vi "New TA Binding.vi"(8 "error in (no error)":errorcluster, 10 "Index (out of array range means creating new)":i32, 11 "Motions in":refnum<class "Motions.lvclass">) -> (0 "error out":errorcluster, 2 "New TA Binding out":T1, 3 "Motions out":refnum<class "Motions.lvclass">)   [LabVIEW 2016, in "Hardware.lvlib" / "Motions.lvlib" / "Motions.lvclass"]
uses:
  <userlib>/Common Components/Hardware/Abstract System/Motions/Motions/Motions.lvclass
  <userlib>/TSPopup/TSPopup.Popup Cluster.ctl
  <userlib>/Common Components/Hardware/Abstract System/Motions/Motions/TA Binding Data.ctl
  <userlib>/Common Components/Hardware/Abstract System/Motions/Motions/Motions.lvclass/Motions.ctl
  <userlib>/Common Components/Hardware/Abstract Hardware/Hardware.lvclass/Hardware.ctl
  <userlib>/TSPopup/TSPopup.Popup Call Parameters.ctl
  <userlib>/TSPopup/TSPopup.Data Type.ctl
  <userlib>/TSPopup/TSPopup.lvclass
  <userlib>/TSPopup/TSPopup.Grid.Cell Info.ctl
  <userlib>/Common Components/Hardware/Abstract Hardware/Read Label.vi
  <userlib>/Common Components/Hardware/Motor/Motor/Motor.lvclass
  C:/Program Files (x86)/National Instruments/LabVIEW 2016/user.lib/Common Components/Hardware/Abstract Hardware/Hardware.lvclass
panel:
  in  "Triggers for Array OR":T2(array[cluster]) {"Triggers for Array AND"."Motor" items=["X", "Y", "Z", "R1", "R3"]}
  in  "Popups":T3 {"Boolean" items=["False", "True"]; "Ring" items=["Enable Motor", "Disable Motor", "Move Motor"]}
  in  "Actions":i32(listbox)
  # "OR"
  # "AND"
  # "Type Sensitive\nPopup"
  # "Boolean Colors"
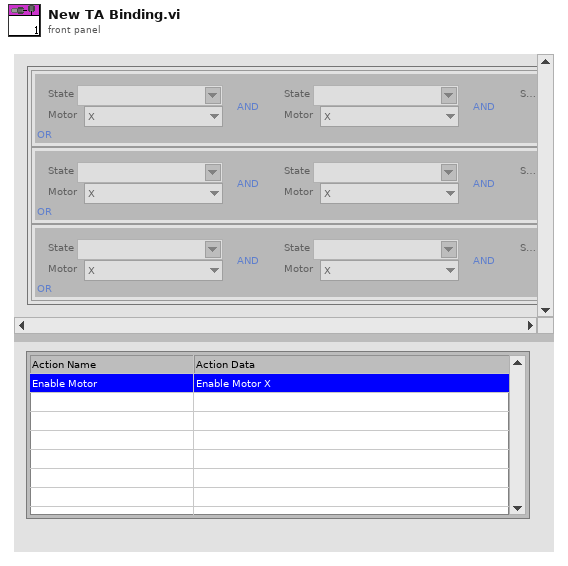
[diagram p1: front panel]
types:
  T1 = typedef "Hardware.lvlib/Motions.lvlib/Motions.lvclass/TA Binding Data.ctl" = cluster{"Triggers":cluster{"Triggers for Array AND":cluster{"Index":u8, "State Name":string}[]}[], "Actions":cluster{"Action Name":string, "Action Data":string}[]}
  T2 = cluster{"Triggers for Array AND":cluster{"Motor":u16, "State":string}[]}[]
  T3 = typedef "TSPopup.lvlib/TSPopup.lvclass/TSPopup.Popup Cluster.ctl" = cluster{"Unknown":bool, "Unknown 2":bool, "String":string, "Integer":i32, "Float":dbl, "Color":u32, "Boolean":u32, "Ring":u32, "Captioned String":cluster{"String":string, "OK":bool, "Cancel":bool}, "Captioned Integer":cluster{"First":i32, "OK":bool, "Cancel":bool}, "Boolean Colors":cluster{"False":cluster{"FG":u32, "BG":u32}, "True":cluster{"FG":u32, "BG":u32}, "T  to  F":cluster{"FG":u32, "BG":u32}, "F  to  T":cluster{"FG":u32, "BG":u32}, "OK":bool, "Cancel":bool}, "2-Int Cluster":cluster{"First":i32, "Second":i32, "OK":bool, "Cancel":bool}, "4-Int Cluster":cluster{"First":i32, "Second":i32, "Third":i32, "Fourth":i32, "OK":bool, "Cancel":bool}, "check":bool}
  T4 = cluster{"Action Name":string, "JSON info":cluster{"path":string, "data type":enum16{"INT", "DBL", "BOOL", "String"}}[], "String Format":string}[]
  T5 = cluster{"Data Types":cluster{"Data Type":string, "Ring Strings":string[]}[]}[]
  T6 = typedef "TSPopup.lvlib/TSPopup.lvclass/TSPopup.Data Type.ctl" = enum16{"Unkown", "NO POPUP", "String", "Integer", "Float", "Color", "Boolean", "Ring", "Captioned String", "Captioned Integer", "Button Color", "2 Int Cluster", "4 Int Cluster", "check"}
  T7 = typedef "TSPopup.lvlib/TSPopup.lvclass/TSPopup.Popup Call Parameters.ctl" = cluster{"Prop Type":T6, "Initial Value":variant, "Caption Strings":string[], "Ring Strings":string[], "Cell Rect":cluster{"left":i16, "top":i16, "right":i16, "bottom":i16}, "Mouse Coords":cluster{"x":i16, "y":i16}, "Call Data":variant}
  T8 = typedef "TSPopup.lvlib/TSPopup.lvclass/TSPopup.Grid.Cell Info.ctl" = cluster{"Tag":string, "Row":i32, "Column":i32, "In Symbol?":bool, "In Data?":bool, "Cell String":string, "Ctl Refnum":refnum<vi>, "Prop Type":T6, "Ring Strings":string[]}
  T9 = cluster{"Data Type":string, "Ring Strings":string[]}[]
  T10 = cluster{"Data Types":cluster{"Data Type":string, "Ring Strings":string[]}[]}
  T11 = typedef "LVPoint32TypeDef.ctl" = cluster{"Horizontal":i32, "Vertical":i32}
  T12 = typedef "LVRowAndColumnTypeDef.ctl" = cluster{"Row":i32, "Column":i32}
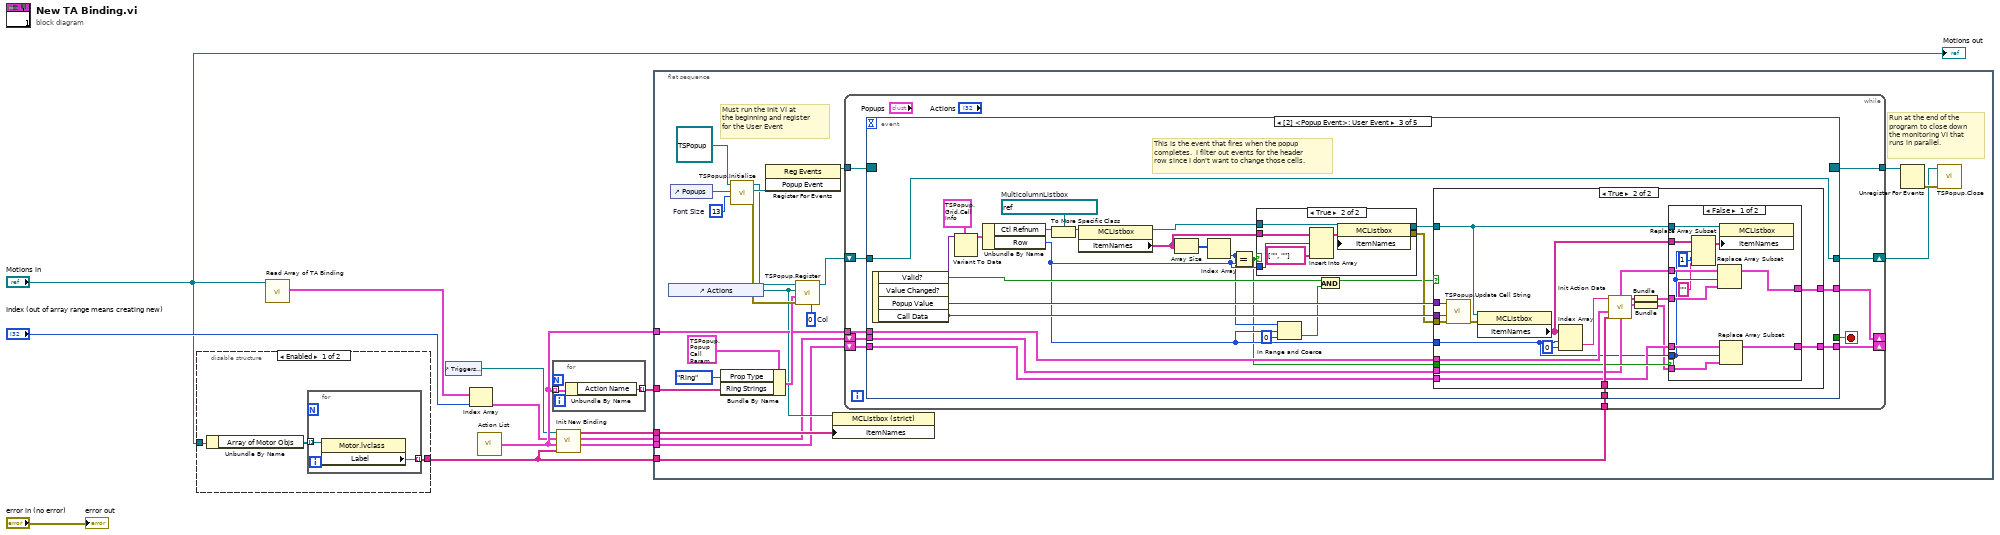
[diagram p0: block diagram]
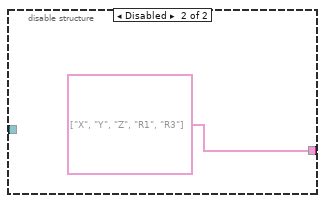
[diagram p2: hidden frame]
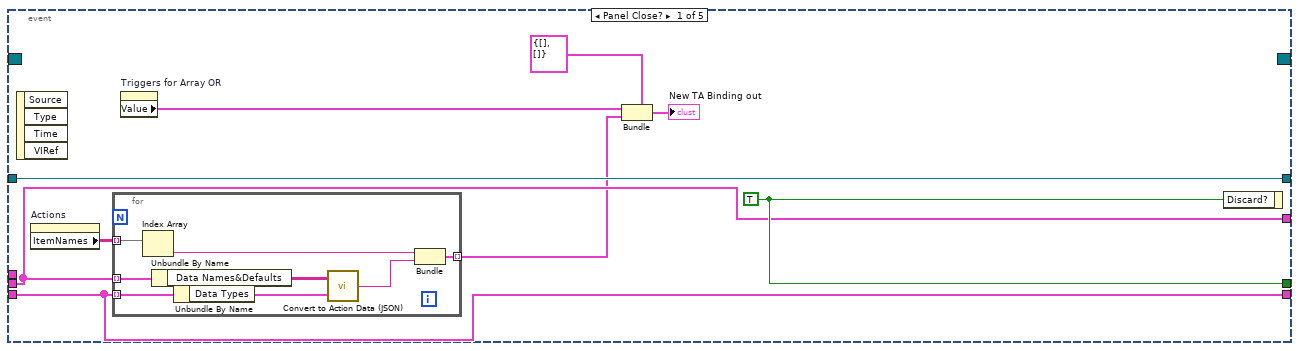
[diagram p3: hidden frame]
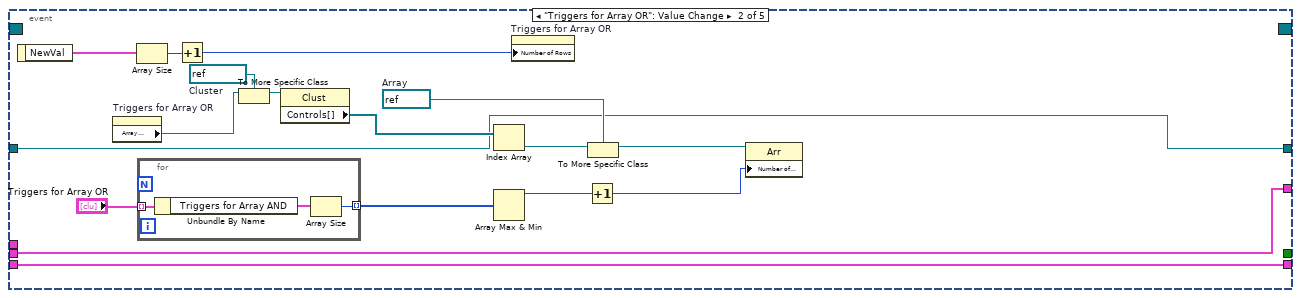
[diagram p4: hidden frame]
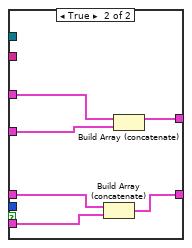
[diagram p7: hidden frame]
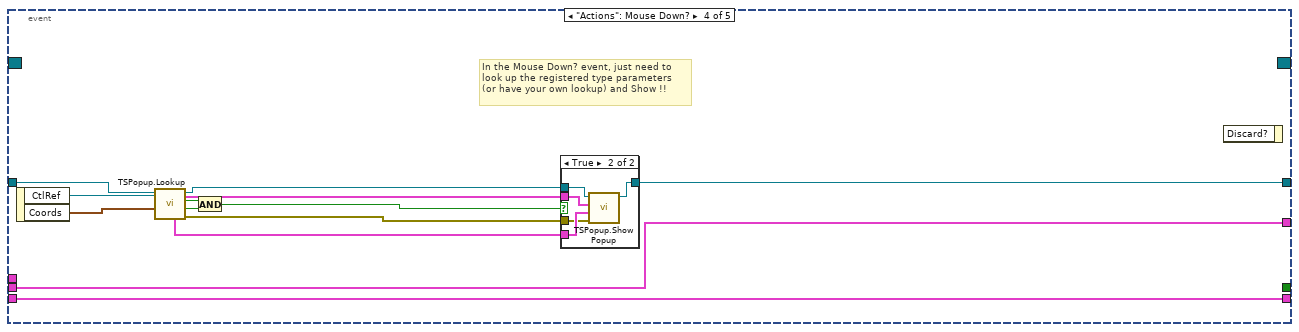
[diagram p8: hidden frame]
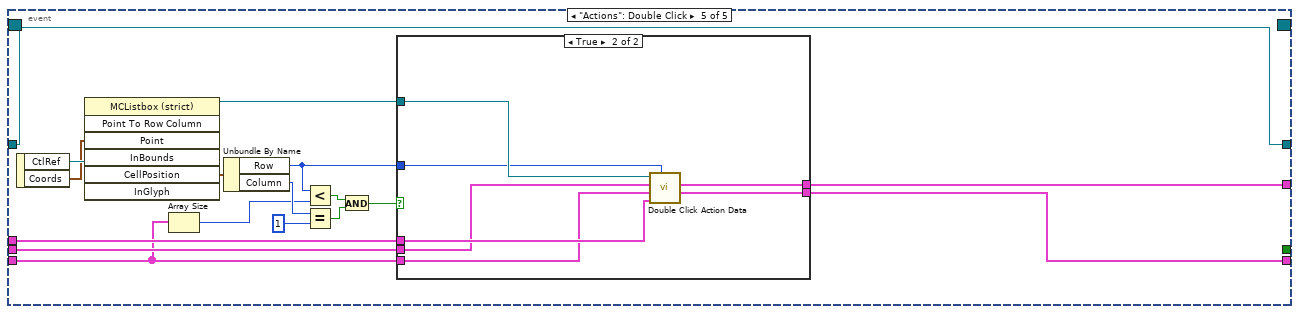
[diagram p10: hidden frame]
diagram:
  n1 = disable-structure shown="Enabled" {
    disable-tunnel: "Motions in" -> [w15 _]
    disable-tunnel: [w13 string[] ["X", "Y", "Z", "R1", "R3"]] -> w2
    frame Enabled {
      n2 = Unbundle By Name(w15) -> ("Array of Motor Objs"=w14:refnum<class "Motor.lvclass">[])
      n3 = for {
        tunnel: w14 -> [w17] mode=indexing
        tunnel: [w16] -> w13 mode=indexing
        n4 = property class="Motor.lvclass"(reference=w17) -> ("Label"=w16:string)  [unwired: 1 in, 2 out]
      }
    }
    frame Disabled {
    }
  }
  n5 = call <userlib>:"Read Array of TA Binding.vi"("Motions in"="Motions in") -> ("Array of TA Binding"=w9:T1[])  [unwired: 9 in, 1 out]
  n6 = control-ref of="Triggers for Array OR"() -> (w7:refnum<vi>)
  n7 = Index Array(array=w9, index="Index (out of array range means creating new)") -> (element=w5:T1)
  n8 = call <userlib>:"Action List.vi"() -> ("Action List"=w11:T4)
  n9 = for {
    tunnel: w11 -> [w20] mode=indexing
    tunnel: [w19] -> w12 mode=indexing
    n10 = Unbundle By Name(w20) -> ("Action Name"=w19:string)
  }
  n11 = call <userlib>:"Init New Binding.vi"("Motor Labels"=w2, "Action List"=w11, "TriggerAction Cluster"=w5, "Triggers Arr Ref"=w7) -> ("Array of Data Types"=w3:T5, "Array of Data Names&Defaults"=w4:cluster{"Data Names&Defaults":string[][]}[], "2-col Arr Actions out"=w6:string[][])  [unwired: 5 in]
  n12 = flat-sequence {
    tunnel: w12 -> [w27]
    tunnel: w11 -> [w26]
    tunnel: w6 -> [w25]
    tunnel: w4 -> [w23]
    tunnel: w3 -> [w22]
    tunnel: w2 -> [w21]
    frame #0 {
      w36 = 0  # Col
      w42 = u32 13  # Font Size
      # "Run at the end of the\nprogram to close down\nthe monitoring VI that\nruns in parallel."
      # "Must run the Init VI at\nthe beginning and register\nfor the User Event"
      n13 = control-ref of="Actions"() -> (w24:refnum<vi>)
      n14 = control-ref of="Popups"() -> (w28:refnum<vi>)
      n15 = Bundle By Name(cluster=T7 {"Prop Type"=enum."Unkown", "Initial Value"=variant, "Caption Strings"=[], "Ring Strings"=[], "Cell Rect"={"left"=0, "top"=0, "right"=0, "bottom"=0}, "Mouse Coords"={"x"=0, "y"=0}, "Call Data"=variant} ("Show Popup (type only)"), "Prop Type"=TSPopup.Data_Type."Ring", "Ring Strings"=w27) -> (w33:T7)
      n16 = call <userlib>:"TSPopup.Initialize.vi"("Font Size"=w42, "Popup Cluster Ref"=w28, "TSPopup in"=refnum<class "TSPopup.lvclass"> refnum) -> ("error out"=w37:errorcluster, "Popup Event"=w41:refnum<user-event>, "TSPopup out"=w31:refnum<class "TSPopup.lvclass">)  [unwired: 6 in]
      n17 = register-events(w41) -> (reference out=w40:refnum<event-registration>)  [unwired: 2 in, 1 out]
      n18 = call <userlib>:"TSPopup.Register.vi"("Col (unwired = all columns)"=w36, "error in (no error)"=w37, "Parameters"=w33, "Ctl Refnum"=w24, "TSPopup in"=w31) -> ("TSPopup out"=w30:refnum<class "TSPopup.lvclass">)  [unwired: 4 in, 2 out]
      n19 = property on="Property Node" class="MCListbox (strict)"(reference=w24, "ItemNames"=w25) -> ()  [unwired: 1 in, 2 out]
      n20 = while {
        tunnel: w40 -> [w53]
        tunnel: [w52] -> w39
        shift-right: [w49] -> w29
        shift-left: w30 -> [w50]
        tunnel: w26 -> [w48]
        shift-right: [w44] -> _
        shift-left: w23 -> [w47]
        shift-right: [w45] -> _
        shift-left: w22 -> [w46]
        tunnel: w21 -> [w43]
        stop <- w51 stop-if-true
        n21 = event shown="[2] <Popup Event>: User Event" {
          selector: w53 -> [_ _ _ _ _]
          dyn-events: [_ _ _ _ _] -> w52
          timeout: _ -> [_ _ _ _ _]
          tunnel: [w62 _ _ _ _] -> w51
          tunnel: w50 -> [w61 w71 w104 w169 w195]
          tunnel: [w61 w71 w104 w167 w195] -> w49
          tunnel: w48 -> [_ _ w103 _ w193]
          tunnel: w47 -> [w57 w73 w95 w166 w192]
          tunnel: w46 -> [w56 w72 w94 w165 w189]
          tunnel: [w56 w72 w92 w165 w191] -> w45
          tunnel: [w57 w73 w93 w166 w190] -> w44
          tunnel: w43 -> [_ _ w102 _ _]
          event Panel Close? {
            w62 = TRUE
            n22 = event-data() -> ()  [unwired: 1 in, 4 out]
            n23 = property on="Actions" class="MCListbox (strict)"() -> ("ItemNames"=w59:string[][])  [unwired: 2 in, 2 out]
            n24 = for {
              tunnel: w59 -> [w70] mode=indexing
              tunnel: [w68] -> w55 mode=indexing
              tunnel: w57 -> [w67] mode=indexing
              tunnel: w56 -> [w66] mode=indexing
              n25 = Index Array(array=w70) -> (element=w69:string)  [unwired: 1 in]
              n26 = Unbundle By Name(w67) -> ("Data Names&Defaults"=w64:string[][])
              n27 = Unbundle By Name(w66) -> ("Data Types"=w63:T9)
              n28 = call <userlib>:"Convert to Action Data (JSON).vi"("Data Types"=w63, "Data Names&Data"=w64) -> ("Action Data (JSON)"=w65:string)
              n29 = Bundle(w69, "Action Data (JSON)"=w65) -> (w68:cluster{string, "Action Data (JSON)":string})  [unwired: 1 in]
            }
            n30 = property on="Triggers for Array OR" class="Arr (strict)"() -> ("Value"=w60:T2)  [unwired: 2 in, 2 out]
            n31 = Bundle(cluster=T1 {"Triggers"=[], "Actions"=[]} ("New TA Binding out"), "Triggers"=w60, "Actions"=w55) -> (→"New TA Binding out":T1)
            n32 = event-data("Discard?"=w62) -> ()  [unwired: 1 in, 1 out]
          }
          event "Triggers for Array OR": Value Change {
            w81 = refnum<vi> refnum  # Array
            w76 = refnum<vi> refnum  # Cluster
            n33 = event-data() -> ("NewVal"=w85:T2)  [unwired: 1 in]
            n34 = property on="Triggers for Array OR" class="Arr (strict)"() -> ("Array Element"=w79:refnum<vi>)  [unwired: 2 in, 2 out]
            n35 = Array Size(array=w85) -> (size(s)=w86:i32)
            n36 = for {
              tunnel: "Triggers for Array OR" -> [w90] mode=indexing
              tunnel: [w88] -> w75 mode=indexing
              n37 = Unbundle By Name(w90) -> ("Triggers for Array AND"=w89:cluster{"Motor":u16, "State":string}[])
              n38 = Array Size(array=w89) -> (size(s)=w88:i32)
            }
            n39 = Increment(x=w86) -> (x+1=w87:i32)
            n40 = To More Specific Class(target class=w76, reference=w79) -> (specific class reference=w77:refnum<vi>)  [unwired: 1 in, 1 out]
            n41 = property class="Clust"(reference=w77) -> ("Controls[]"=w78:refnum<vi>[])  [unwired: 1 in, 2 out]
            n42 = Index Array(array=w78) -> (element=w80:refnum<vi>)  [unwired: 1 in]
            n43 = Array Max & Min(array=w75) -> (max value=w83:i32)  [unwired: 3 out]
            n44 = property on="Triggers for Array OR" class="Arr (strict)"("Number of Rows"=w87) -> ()  [unwired: 2 in, 2 out]
            n45 = Increment(x=w83) -> (x+1=w84:i32)
            n46 = To More Specific Class(target class=w81, reference=w80) -> (specific class reference=w82:refnum<vi>)  [unwired: 1 in, 1 out]
            n47 = property class="Arr"(reference=w82, "Number of Columns"=w84) -> ()  [unwired: 1 in, 2 out]
          }
          event User Event {
            w109 = refnum<vi> refnum  # MulticolumnListbox
            # "This is the event that fires when the popup\ncompletes.  I filter out events for the header\nrow since I don't want to change those cells."
            n48 = event-data() -> ("Valid?"=w116:bool, "Popup Value"=w115:variant, "Call Data"=w114:variant)  [unwired: 1 in, 1 out]
            n49 = Variant To Data(type=T8 {"Tag"="", "Row"=0, "Column"=0, "In Symbol?"=FALSE, "In Data?"=FALSE, "Cell String"="", "Ctl Refnum"=refnum, "Prop Type"=enum."Unkown", "Ring Strings"=[]} ("Cell Info (type only)"), Variant=w114) -> (data=w113:T8)  [unwired: 1 in, 1 out]
            n50 = Unbundle By Name(w113) -> ("Ctl Refnum"=w111:refnum<vi>, "Row"=w100:i32)
            n51 = To More Specific Class(target class=w109, reference=w111) -> (specific class reference=w110:refnum<vi>)  [unwired: 1 in, 1 out]
            n52 = property class="MCListbox"(reference=w110) -> (reference out=w106:refnum<vi>, "ItemNames"=w107:string[][])  [unwired: 1 in, 1 out]
            n53 = Array Size(array=w107) -> (size(s)=w108:i32[])
            n54 = Index Array(array=w108) -> (element=w99:i32)  [unwired: 1 in]
            n55 = Equal?(x=w99, y=w100) -> (x = y?=w96:bool)
            n56 = case shown="True" w96 {
              tunnel: w107 -> [_ w124]
              tunnel: w100 -> [_ w123]
              tunnel: w106 -> [w117 w121]
              tunnel: [_ w119] -> w105
              tunnel: [w117 w118] -> w91
              frame False {
              }
              frame True {
                n57 = Insert Into Array(array=w124, index (row)=w123, new element=string[] ["", ""] ("new element/subarray")) -> (w120:string[][])  [unwired: 1 in]
                n58 = property class="MCListbox"(reference=w121, "ItemNames"=w120) -> (reference out=w118:refnum<vi>, error out=w119:errorcluster)  [unwired: 1 in]
              }
            }
            n59 = In Range and Coerce(upper limit=w99, x=w100, lower limit=0) -> (In Range?=w97:bool)  [unwired: 1 out]
            n60 = And(x=w116, y=w97) -> (x .and. y?=w98:bool)
            n61 = case shown="True" w98 {
              tunnel: w115 -> [_ w145]
              tunnel: w114 -> [_ w146]
              tunnel: w105 -> [_ w144]
              tunnel: w100 -> [_ w132]
              tunnel: w103 -> [_ w140]
              tunnel: w102 -> [_ w139]
              tunnel: w96 -> [_ w138]
              tunnel: w95 -> [w126 w137]
              tunnel: w94 -> [w125 w136]
              tunnel: [w126 w134] -> w93
              tunnel: [w125 w133] -> w92
              tunnel: w91 -> [_ w128]
              frame False {
              }
              frame True {
                n62 = call <userlib>:"TSPopup.Update Cell String.vi"("error in (no error)"=w144, "Call Data (must be Cell Info cluster)"=w146, "Popup Value"=w145) -> ("error out"=w143:errorcluster)  [unwired: 8 in]
                n63 = property class="MCListbox"(reference=w128, error in=w143) -> ("ItemNames"=w127:string[][])  [unwired: 2 out]
                n64 = Index Array(array=w127, index (row)=w132, index (col)=0 ("disabled index (col)")) -> (element=w141:string)
                n65 = call <userlib>:"Init Action Data.vi"("Motor Labels"=w139, "Action List"=w140, "Action Name"=w141) -> ("Data Types"=w130:T9, "Data Names&Defaults"=w135:string[][])  [unwired: 7 in]
                n66 = Bundle("Data Names&Defaults"=w135) -> (w131:cluster{"Data Names&Defaults":string[][]})  [unwired: 1 in]
                n67 = Bundle("Data Types"=w130) -> (w129:T10)  [unwired: 1 in]
                n68 = case shown="False" w138 {
                  tunnel: w137 -> [w158 w164]
                  tunnel: w136 -> [w155 w163]
                  tunnel: w131 -> [w156 w160]
                  tunnel: w129 -> [w153 w159]
                  tunnel: [w157 w162] -> w134
                  tunnel: [w154 w161] -> w133
                  tunnel: w132 -> [w150 _]
                  tunnel: w128 -> [w152 _]
                  tunnel: w127 -> [w151 _]
                  frame False {
                    n69 = Replace Array Subset(array=w151, new element="" ("new element/subarray"), index (row)=w150, index (col)=1 ("disabled index (col)")) -> (w149:string[][])
                    n70 = Replace Array Subset(array=w158, new element=w156, index=w150) -> (w157:cluster{"Data Names&Defaults":string[][]}[])
                    n71 = Replace Array Subset(array=w155, new element=w153, index=w150) -> (w154:T5)
                    n72 = property class="MCListbox"(reference=w152, "ItemNames"=w149) -> ()  [unwired: 1 in, 2 out]
                  }
                  frame True {
                    n73 = Build Array (concatenate)(w163, w159) -> (w161:T5)
                    n74 = Build Array (concatenate)(w164, w160) -> (w162:cluster{"Data Names&Defaults":string[][]}[])
                  }
                }
              }
            }
          }
          event "Actions": Mouse Down? {
            # "In the Mouse Down? event, just need to\nlook up the registered type parameters\n(or have your own lookup) and Show !!"
            n75 = event-data() -> ("CtlRef"=w170:refnum<vi>, "Coords"=w177:T11)  [unwired: 1 in]
            n76 = call <userlib>:"TSPopup.Lookup.vi"("Point"=w177, "Ctl Refnum"=w170, "TSPopup in"=w169) -> ("error out"=w171:errorcluster, "In Bounds?"=w175:bool, "Found"=w176:bool, "TSPopup out"=w168:refnum<class "TSPopup.lvclass">, "Cell Info (Call data)"=w172:T8, "Popup Parameters"=w173:T7)  [unwired: 3 in]
            n77 = And(x=w176, y=w175) -> (x .and. y?=w174:bool)
            n78 = case shown="True" w174 {
              tunnel: w173 -> [_ w183]
              tunnel: w172 -> [_ w182]
              tunnel: w171 -> [_ w181]
              tunnel: w168 -> [w178 w180]
              tunnel: [w178 w179] -> w167
              frame False {
              }
              frame True {
                n79 = call <userlib>:"TSPopup.Show Popup.vi"("error in (no error)"=w181, "Call Data (ignore if empty)"=w182, "Popup Parameters"=w183, "TSPopup in"=w180) -> ("TSPopup out"=w179:refnum<class "TSPopup.lvclass">)  [unwired: 6 in, 1 out]
              }
            }
            n80 = event-data() -> ()  [unwired: 2 in, 1 out]
          }
          event "Actions": Double Click {
            n81 = event-data() -> ("CtlRef"=w200:refnum<vi>, "Coords"=w199:T11)  [unwired: 1 in]
            n82 = invoke class="MCListbox (strict)" method="Point To Row Column"(reference=w200, "Point"=w199) -> (reference out=w194:refnum<vi>, "CellPosition"=w198:T12)  [unwired: 5 in, 5 out]
            n83 = Array Size(array=w189) -> (size(s)=w184:i32)
            n84 = Unbundle By Name(w198) -> ("Row"=w188:i32, "Column"=w197:i32)
            n85 = Less?(x=w188, y=w184) -> (x < y?=w187:bool)
            n86 = Equal?(x=w197, y=1) -> (x = y?=w186:bool)
            n87 = And(x=w187, y=w186) -> (x .and. y?=w185:bool)
            n88 = case shown="True" w185 {
              tunnel: w188 -> [_ w208]
              tunnel: w194 -> [_ w209]
              tunnel: w193 -> [_ w207]
              tunnel: w192 -> [w202 w206]
              tunnel: w189 -> [w201 w205]
              tunnel: [w201 w204] -> w191
              tunnel: [w202 w203] -> w190
              frame False {
              }
              frame True {
                n89 = call <userlib>:"Double Click Action Data.vi"("Row"=w208, "Action List"=w207, "Array of Data Types in"=w205, "Array of Data Names&Defaults in"=w206, "MCListbox Ref"=w209) -> ("Array of Data Types out"=w204:T5, "Array of Data Names&Defaults out"=w203:cluster{"Data Names&Defaults":string[][]}[])  [unwired: 5 in]
              }
            }
          }
        }
      }
      n90 = Unregister For Events(event registration refnum=w39) -> (error out=w38:errorcluster)  [unwired: 1 in]
      n91 = call <userlib>:"TSPopup.Close.vi"("error in (no error)"=w38, "TSPopup in"=w29) -> ()  [unwired: 8 in, 2 out]
    }
  }
  "error out" <- "error in (no error)"
  "Motions out" <- "Motions in"
